vi "setUp.vi"(8 "error in (no error)":errorcluster, 11 "reference in":refnum<class "testcase-CSMGlobalLog.lvclass">) -> (0 "error out":errorcluster, 3 "reference out":refnum<class "testcase-CSMGlobalLog.lvclass">)   [LabVIEW 2017, in "testcase-CSMGlobalLog.lvclass"]
doc: "setUp runs prior to the test method during test execution. Use this method to initialize any object data required by your tests."
uses:
  testcase-CSMGlobalLog.lvclass
  C:/Program Files (x86)/National Instruments/LabVIEW 2017/vi.lib/addons/_JKI Toolkits/VI Tester/TestCase.llb/TestCase.lvclass
  <vilib>/addons/_JKI Toolkits/VI Tester/TestCase.llb/TestCase.lvclass
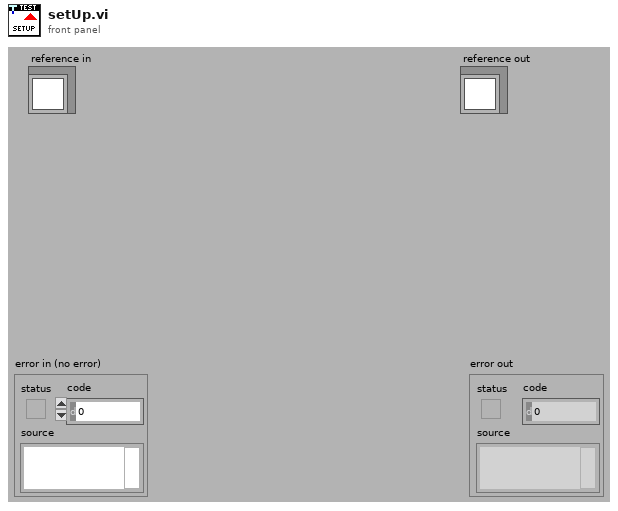
[diagram p1: front panel]
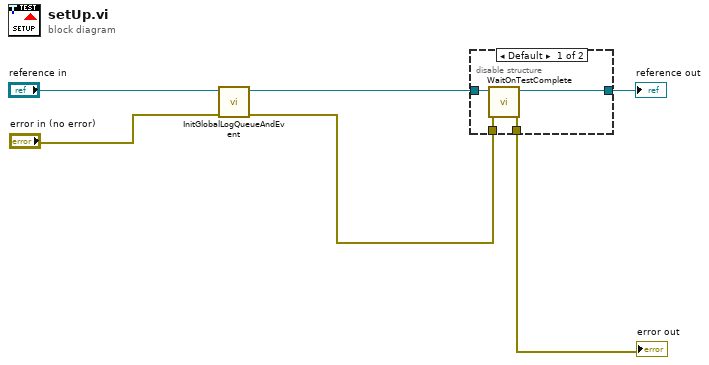
[diagram p0: block diagram]
diagram:
  n1 = call "InitGlobalLogQueueAndEvent.vi"("error in (no error)"="error in (no error)", "TestCase in"="reference in") -> ("error out"=w2:errorcluster, "TestCase out"=w1:refnum<class "testcase-CSMGlobalLog.lvclass">)  [unwired: 6 in, 2 out]
  n2 = disable-structure shown="Default" {
    disable-tunnel: w2 -> [w10 w11]
    disable-tunnel: [w9 w11] -> w6
    disable-tunnel: [w8 w12] -> w5
    disable-tunnel: w1 -> [w7 w12]
    frame condition #0 (active) {
      n3 = call <vilib>:"WaitOnTestComplete.vi"("error in (no error)"=w10, "TestCase in"=w7) -> ("error out"=w9:errorcluster, "TestCase out"=w8:refnum<class "testcase-CSMGlobalLog.lvclass">)  [unwired: 8 in]
    }
    frame condition #1 {
    }
  }
  "error out" <- w6
  "reference out" <- w5
